vi "IMGHDR_write.vi"(8 "error in (no error)":errorcluster, 10 "IMGHDR":T1, 11 "refnum in":refnum<file>) -> (0 "error out":errorcluster, 3 "refnum out":refnum<file>)   [LabVIEW 2012]
uses:
  TTTR_data_headers/IMGHDR.ctl
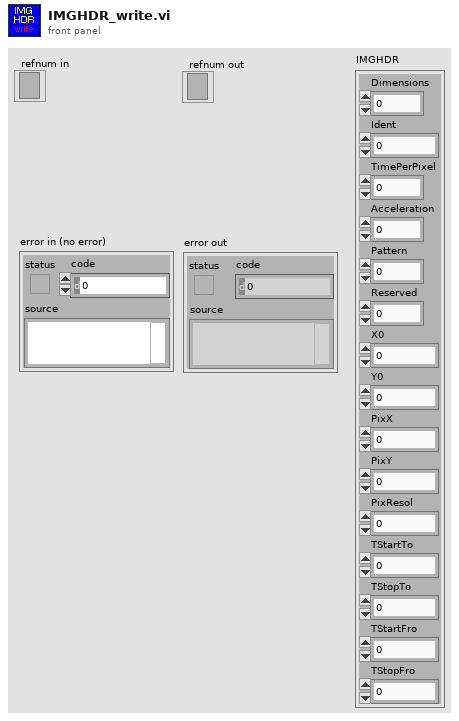
[diagram p1: front panel]
types:
  T1 = typedef "IMGHDR.ctl" = cluster{"Dimensions":i32, "Ident":i32, "TimePerPixel":i32, "Acceleration":i32, "Pattern":i32, "Reserved":i32, "X0":sgl, "Y0":sgl, "PixX":i32, "PixY":i32, "PixResol":sgl, "TStartTo":sgl, "TStopTo":sgl, "TStartFro":sgl, "TStopFro":sgl}
  T2 = enum16{"big-endian, network order", "native, host order", "little-endian"}
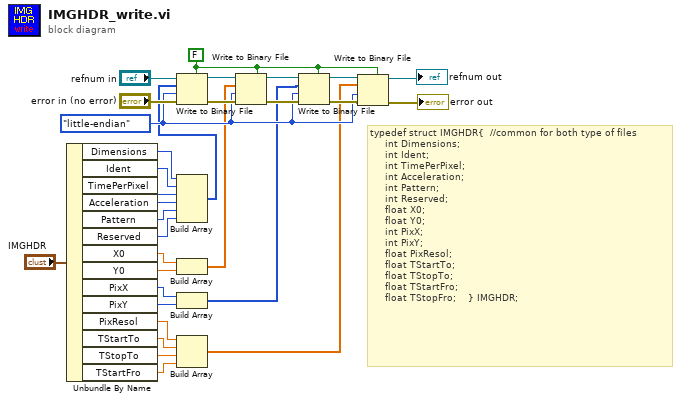
[diagram p0: block diagram]
diagram:
  w19 = FALSE ("prepend array or string size? (T)")
  w21 = T2."little-endian" ("byte order (0:big-endian, network order)")
  # "typedef struct IMGHDR{\t\t//common for both type of files\n  \t\t\tint Dimensions;\n  \t\t\tint Ident;\n  \t\t\tint TimePerPixel;\n  \t\t\tint Acceleration;\n  \t\t\tint Pattern;\n  \t\t\tint Reserved;\n  \t\t\tfloat X0;\n  \t\t\tfloat Y0;\n  \t\t\tint PixX;\n  \t\t\tint PixY;\n  \t\t\tfloat PixResol;\n  \t\t\tfloat TStartTo;\n  \t\t\tfloat TStopTo;\n  \t\t\tfloat TStartFro;\n  \t\t\tfloat TStopFro;    } IMGHDR;"
  n1 = Unbundle By Name("IMGHDR") -> ("Dimensions"=w5:i32, "Ident"=w6:i32, "TimePerPixel"=w7:i32, "Acceleration"=w8:i32, "Pattern"=w9:i32, "Reserved"=w10:i32, "X0"=w11:sgl, "Y0"=w12:sgl, "PixX"=w13:i32, "PixY"=w14:i32, "PixResol"=w15:sgl, "TStartTo"=w16:sgl, "TStopTo"=w17:sgl, "TStartFro"=w18:sgl)
  n2 = Build Array(w5, w6, w7, w8, w9, w10) -> (w4:i32[])
  n3 = Write to Binary File(file (use dialog)="refnum in", data=w4, error in="error in (no error)", 5:w19, 9:w21) -> (refnum out=w28:refnum<file>, error out=w29:errorcluster)  [unwired: 1 in, 1 out]
  n4 = Build Array(w11, w12) -> (w3:sgl[])
  n5 = Build Array(w13, w14) -> (w2:i32[])
  n6 = Build Array(w15, w16, w17, w18) -> (w1:sgl[])
  n7 = Write to Binary File(file (use dialog)=w28, data=w3, error in=w29, 5:w19, 9:w21) -> (refnum out=w26:refnum<file>, error out=w27:errorcluster)  [unwired: 1 in, 1 out]
  n8 = Write to Binary File(file (use dialog)=w26, data=w2, error in=w27, 5:w19, 9:w21) -> (refnum out=w22:refnum<file>, error out=w23:errorcluster)  [unwired: 1 in, 1 out]
  n9 = Write to Binary File(file (use dialog)=w22, data=w1, error in=w23, 5:w19, 9:w21) -> (refnum out=→"refnum out":refnum<file>, error out=→"error out":errorcluster)  [unwired: 1 in, 1 out]
